vi "Check Data Size (word).vi"(1 "error in (no error)":errorcluster, 2 "rect":T1, 3 "depth":u8, 4 "flattened image data":u8[](array[numeric])) -> (0 "error out":errorcluster)   [LabVIEW 2010, in "NI_ReportGenerationToolkit.lvlib"]
doc: "Checks the flattened data to see if the size of the data in bytes is what we expect it to be based on its bounds and depth."
uses:
  <vilib>/addons/_office/NI_ReportGenerationToolkit.lvlib
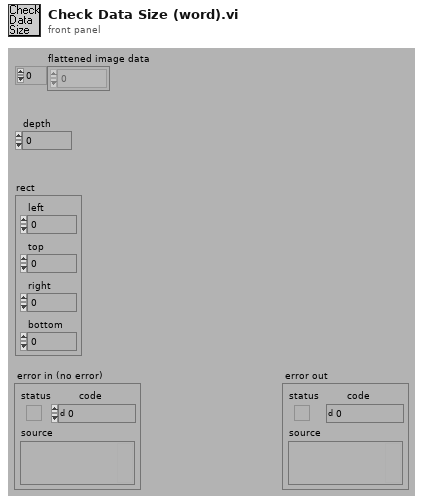
[diagram p1: front panel]
types:
  T1 = cluster{"left":i16, "top":i16, "right":i16, "bottom":i16}
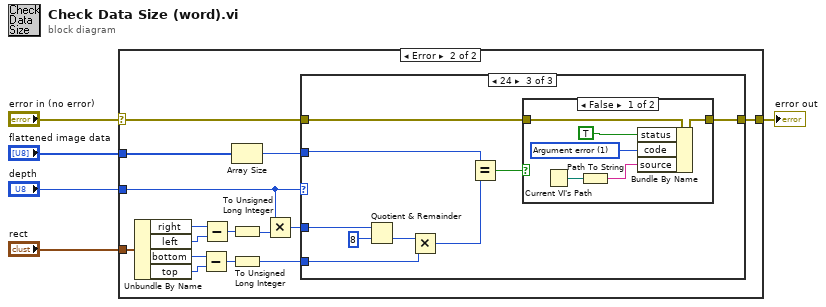
[diagram p0: block diagram]
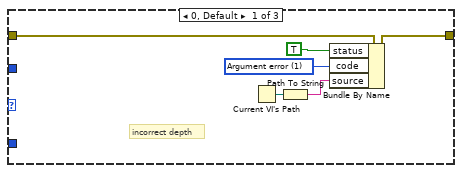
[diagram p3: hidden frame]
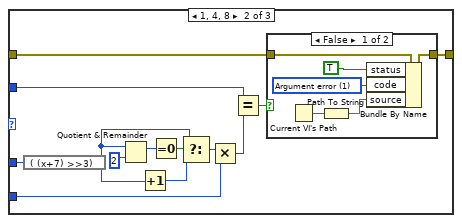
[diagram p4: hidden frame]
diagram:
  n1 = case shown="Error" "error in (no error)" {
    selector: "error in (no error)" -> [w6 w8]
    tunnel: "depth" -> [_ w18]
    tunnel: "rect" -> [_ w17]
    tunnel: [w6 w12] -> w3
    tunnel: "flattened image data" -> [_ w11]
    frame No Error {
    }
    frame Error {
      n2 = Unbundle By Name(w17) -> ("right"=w13:i16, "left"=w7:i16, "bottom"=w16:i16, "top"=w15:i16)
      n3 = Subtract(x=w16, y=w15) -> (x-y=w19:i16)
      n4 = Subtract(x=w13, y=w7) -> (x-y=w14:i16)
      n5 = Array Size(array=w11) -> (size(s)=w21:i32)
      n6 = To Unsigned Long Integer(number=w14) -> (unsigned 32bit integer=w10:u32)
      n7 = To Unsigned Long Integer(number=w19) -> (unsigned 32bit integer=w9:u32)
      n8 = Multiply(x=w18, y=w10) -> (x*y=w20:u32)
      n9 = case shown="24" w18 {
        tunnel: w8 -> [w23 w34 w54]
        tunnel: [w22 w38 w53] -> w12
        tunnel: w9 -> [_ w37 w49]
        tunnel: w20 -> [_ w36 w52]
        tunnel: w21 -> [_ w35 w56]
        frame 0, Default {
          w26 = 1 items=["No error", "Argument error", "Memory is full", "Out of zone", "End of file", "File already open", "Generic file I/O error", "File not found", "File permission error", "Disk is full", "Duplicate path", "Too many files open", "System feature not enabled", "Resource file not found", "Cannot add resource", "Resource not found", "Image not found", "Image memory error", "Pen does not exist", "Config type invalid", "Config token not found", "Config parse error", "Config memory error", "Bad external code format", "Bad external code offset", "External code not present", "Null window", "Destroy window error", "Null menu", "Print aborted", "Bad print record", "Print driver error", "Windows error during printing", "Memory error during printing", "Print dialog error", "Generic print error", "Invalid device refnum", "Device not found", "Device parameter error", "Device unit error", "Cannot open device", "Device call aborted", "Generic error", "Cancelled by user", "Object ID too low", "Object ID too high", "Object not in heap", "Unknown heap", "Unknown object (invalid DefProc)", "Unknown object (DefProc not in table)", "Message out of range", "Invalid (null) method", "Unknown message", "Manager call not supported", "Bad address", "Network operation in progress", "Network operation timed out", "Connection is busy", "Network attribute not supported", "Network error", "Address in use", "System out of memory", "Connection aborted", "Connection refused", "Not connected", "Already connected", "Connection closed", "Initialization error (interapplication manager)", "Bad occurrence", "Wait on unbound occurrence handler", "Occurrence queue overflow", "Datalog type conflict", "Unused", "Unrecognized type (interapplication manager)", "Memory corrupt", "Failed to make temporary DLL", "Old CIN version", "Drag socket not found", "Failed to load drop-object", "Failed to register OLE object", "Failed to release OLE object", "Format specifier type mismatch", "Unknown format specifier", "Too few format specifiers", "Too many format specifiers", "Scan failed", "Newer CIN version", "Error converting to variant", "Runtime menu error", "Password tampered", "Variant attribute not found", "Incompatible variant data type", "Event data is not available", "Event Store is not present", "Occurrence is not found", "Event Queue is not created", "Event info is not available", "Refnum passed is NULL", "Error retrieving Class GUID", "Error retrieving CoClass GUID", "Error retrieving TypeLib GUID.", "Bad built application magic bytes.", "Specific driver is different from the specific driver associated with the Logical Name.", "There is no session opened to the class driver.", "Max Error", "MAX - Error with config objects", "MAX - Error loading configuration", "MAX - Group not supported"]
          # "incorrect depth"
          n10 = Current VI's Path() -> (path=w25:path)
          n11 = Path To String(path=w25) -> (string=w24:string)
          n12 = Bundle By Name(cluster=w23, "status"=TRUE, "code"=w26, "source"=w24) -> (w22:errorcluster)
        }
        frame 1, 4, 8 {
          n13 = expression code="(\t(x+7) >>3)"(w36) -> (w28:u32)
          n14 = Quotient & Remainder(x=w28, y=u32 2 ("x")) -> (x-y*floor(x/y)=w33:u32)  [unwired: 1 out]
          n15 = Increment(x=w28) -> (x+1=w32:u32)
          n16 = Equal To 0?(x=w33) -> (x = 0?=w31:bool)
          n17 = Select(t=w28, s=w31, f=w32) -> (s? t:f=w30:u32)
          n18 = Multiply(x=w30, y=w37) -> (x*y=w40:u32)
          n19 = Equal?(x=w35, y=w40) -> (x = y?=w39:bool)
          n20 = case shown="False" w39 {
            tunnel: w34 -> [w42 w47]
            tunnel: [w41 w47] -> w38
            frame False {
              w45 = 1 items=["No error", "Argument error", "Memory is full", "Out of zone", "End of file", "File already open", "Generic file I/O error", "File not found", "File permission error", "Disk is full", "Duplicate path", "Too many files open", "System feature not enabled", "Resource file not found", "Cannot add resource", "Resource not found", "Image not found", "Image memory error", "Pen does not exist", "Config type invalid", "Config token not found", "Config parse error", "Config memory error", "Bad external code format", "Bad external code offset", "External code not present", "Null window", "Destroy window error", "Null menu", "Print aborted", "Bad print record", "Print driver error", "Windows error during printing", "Memory error during printing", "Print dialog error", "Generic print error", "Invalid device refnum", "Device not found", "Device parameter error", "Device unit error", "Cannot open device", "Device call aborted", "Generic error", "Cancelled by user", "Object ID too low", "Object ID too high", "Object not in heap", "Unknown heap", "Unknown object (invalid DefProc)", "Unknown object (DefProc not in table)", "Message out of range", "Invalid (null) method", "Unknown message", "Manager call not supported", "Bad address", "Network operation in progress", "Network operation timed out", "Connection is busy", "Network attribute not supported", "Network error", "Address in use", "System out of memory", "Connection aborted", "Connection refused", "Not connected", "Already connected", "Connection closed", "Initialization error (interapplication manager)", "Bad occurrence", "Wait on unbound occurrence handler", "Occurrence queue overflow", "Datalog type conflict", "Unused", "Unrecognized type (interapplication manager)", "Memory corrupt", "Failed to make temporary DLL", "Old CIN version", "Drag socket not found", "Failed to load drop-object", "Failed to register OLE object", "Failed to release OLE object", "Format specifier type mismatch", "Unknown format specifier", "Too few format specifiers", "Too many format specifiers", "Scan failed", "Newer CIN version", "Error converting to variant", "Runtime menu error", "Password tampered", "Variant attribute not found", "Incompatible variant data type", "Event data is not available", "Event Store is not present", "Occurrence is not found", "Event Queue is not created", "Event info is not available", "Refnum passed is NULL", "Error retrieving Class GUID", "Error retrieving CoClass GUID", "Error retrieving TypeLib GUID.", "Bad built application magic bytes.", "Specific driver is different from the specific driver associated with the Logical Name.", "There is no session opened to the class driver.", "Max Error", "MAX - Error with config objects", "MAX - Error loading configuration", "MAX - Group not supported"]
              n21 = Current VI's Path() -> (path=w44:path)
              n22 = Path To String(path=w44) -> (string=w43:string)
              n23 = Bundle By Name(cluster=w42, "status"=TRUE, "code"=w45, "source"=w43) -> (w41:errorcluster)
            }
            frame True {
            }
          }
        }
        frame 24 {
          n24 = Quotient & Remainder(x=w52, y=u32 8) -> (floor(x/y)=w50:u32)  [unwired: 1 out]
          n25 = Multiply(x=w50, y=w49) -> (x*y=w48:u32)
          n26 = Equal?(x=w56, y=w48) -> (x = y?=w55:bool)
          n27 = case shown="False" w55 {
            tunnel: w54 -> [w58 w63]
            tunnel: [w57 w63] -> w53
            frame False {
              w61 = 1 items=["No error", "Argument error", "Memory is full", "Out of zone", "End of file", "File already open", "Generic file I/O error", "File not found", "File permission error", "Disk is full", "Duplicate path", "Too many files open", "System feature not enabled", "Resource file not found", "Cannot add resource", "Resource not found", "Image not found", "Image memory error", "Pen does not exist", "Config type invalid", "Config token not found", "Config parse error", "Config memory error", "Bad external code format", "Bad external code offset", "External code not present", "Null window", "Destroy window error", "Null menu", "Print aborted", "Bad print record", "Print driver error", "Windows error during printing", "Memory error during printing", "Print dialog error", "Generic print error", "Invalid device refnum", "Device not found", "Device parameter error", "Device unit error", "Cannot open device", "Device call aborted", "Generic error", "Cancelled by user", "Object ID too low", "Object ID too high", "Object not in heap", "Unknown heap", "Unknown object (invalid DefProc)", "Unknown object (DefProc not in table)", "Message out of range", "Invalid (null) method", "Unknown message", "Manager call not supported", "Bad address", "Network operation in progress", "Network operation timed out", "Connection is busy", "Network attribute not supported", "Network error", "Address in use", "System out of memory", "Connection aborted", "Connection refused", "Not connected", "Already connected", "Connection closed", "Initialization error (interapplication manager)", "Bad occurrence", "Wait on unbound occurrence handler", "Occurrence queue overflow", "Datalog type conflict", "Unused", "Unrecognized type (interapplication manager)", "Memory corrupt", "Failed to make temporary DLL", "Old CIN version", "Drag socket not found", "Failed to load drop-object", "Failed to register OLE object", "Failed to release OLE object", "Format specifier type mismatch", "Unknown format specifier", "Too few format specifiers", "Too many format specifiers", "Scan failed", "Newer CIN version", "Error converting to variant", "Runtime menu error", "Password tampered", "Variant attribute not found", "Incompatible variant data type", "Event data is not available", "Event Store is not present", "Occurrence is not found", "Event Queue is not created", "Event info is not available", "Refnum passed is NULL", "Error retrieving Class GUID", "Error retrieving CoClass GUID", "Error retrieving TypeLib GUID.", "Bad built application magic bytes.", "Specific driver is different from the specific driver associated with the Logical Name.", "There is no session opened to the class driver.", "Max Error", "MAX - Error with config objects", "MAX - Error loading configuration", "MAX - Group not supported"]
              n28 = Current VI's Path() -> (path=w60:path)
              n29 = Path To String(path=w60) -> (string=w59:string)
              n30 = Bundle By Name(cluster=w58, "status"=TRUE, "code"=w61, "source"=w59) -> (w57:errorcluster)
            }
            frame True {
            }
          }
        }
      }
    }
  }
  "error out" <- w3
